vi "QR Decomposition.vi"   [LabVIEW 2010, in "NI_AALPro.lvlib"]
doc: "Performs the QR decomposition of <B>A</B> with or without column pivoting. Wire data to the <B>A</B> input to determine the polymorphic instance to use or manually select the instance."
uses:
  NI_AALPro.lvlib
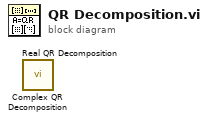
[diagram p0: block diagram]
diagram:
  n1 = call "Complex QR Decomposition.vi"() -> ()  [unwired: 8 in, 4 out]
  n2 = call "Real QR Decomposition.vi"() -> ()  [unwired: 8 in, 4 out]
